vi "Config files dialogue Window.vi"(7 "Colour":u32(colorbox)=16777225, 8 "error in (no error)":errorcluster, 9 "Caption-Left button (Cancel)":string, 10 "Caption-Right button (OK)":string, 11 "Message string":string) -> (0 "error out":errorcluster, 1 "Cancelled (Left button pressed)":bool)   [LabVIEW 2020]
doc: "Use this template to create a dialog box with event handling."
uses:
  <vilib>/Utility/miscctls.llb/LVPointTypeDef.ctl
  Global Variables/General Globals.vi
panel:
  in  "Left Button":bool
  in  "Rigth Button":bool
  out "Message":string
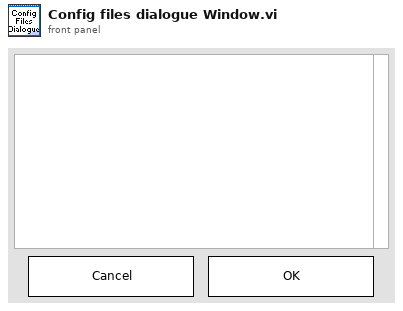
[diagram p1: front panel]
types:
  T1 = typedef "LVPointTypeDef.ctl" = cluster{"Horizontal":i16, "Vertical":i16}
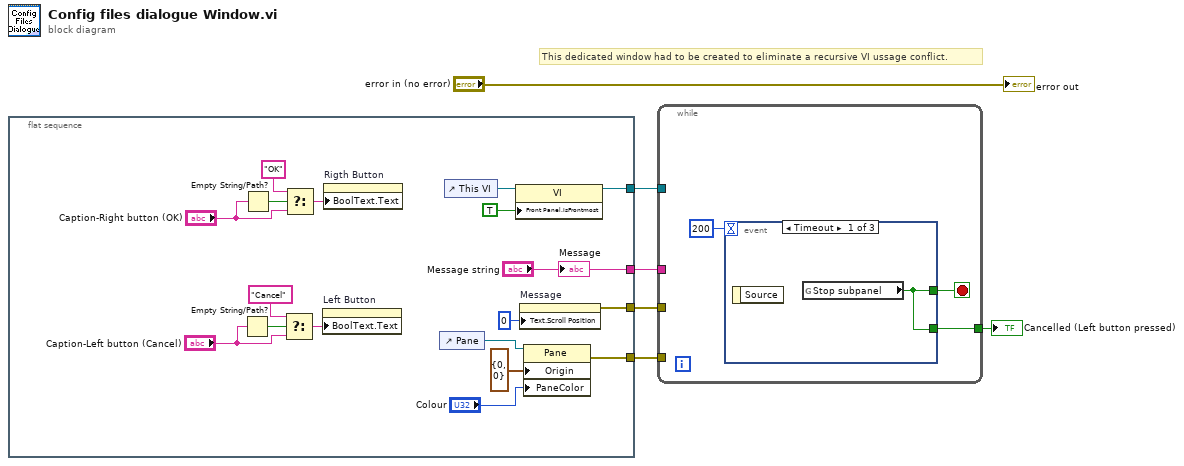
[diagram p0: block diagram]
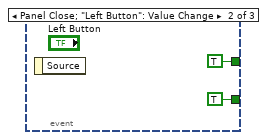
[diagram p2: hidden frame]
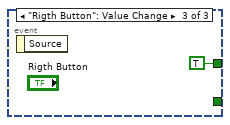
[diagram p3: hidden frame]
diagram:
  # "This dedicated window had to be created to eliminate a recursive VI ussage conflict."
  n1 = flat-sequence {
    tunnel: ["Message string"] -> w6
    tunnel: [w22] -> w5
    tunnel: [w19] -> w4
    tunnel: [w17] -> w3
    frame #0 {
      n2 = Empty String/Path?(string/path="Caption-Left button (Cancel)") -> (empty?=w10:bool)
      n3 = Empty String/Path?(string/path="Caption-Right button (OK)") -> (empty?=w14:bool)
      n4 = Select(t="Cancel", s=w10, f="Caption-Left button (Cancel)") -> (s? t:f=w9:string)
      n5 = Select(t="OK", s=w14, f="Caption-Right button (OK)") -> (s? t:f=w12:string)
      n6 = property on="Left Button" class="Bool"("BoolText.Text"=w9) -> ()  [unwired: 2 in, 2 out]
      n7 = property on="Rigth Button" class="Bool"("BoolText.Text"=w12) -> ()  [unwired: 2 in, 2 out]
      n8 = control-ref of="Pane"() -> (w16:refnum<vi>)
      n9 = control-ref of="This VI"() -> (w20:refnum<vi>)
      n10 = property on="Property Node" class="VI"(reference=w20, "Front Panel.IsFrontmost"=TRUE ("Front Panel Window:Is Frontmost")) -> (reference out=w19:refnum<vi>)  [unwired: 1 in, 1 out]
      n11 = property on="Message" class="Str"("Text.Scroll Position"=u32 0) -> (error out=w22:errorcluster)  [unwired: 2 in, 1 out]
      n12 = property class="Pane"(reference=w16, "Origin"=T1 {"Horizontal"=0, "Vertical"=0}, "PaneColor"="Colour") -> (error out=w17:errorcluster)  [unwired: 1 in, 1 out]
      "Message" <- "Message string"
    }
  }
  n13 = while {
    tunnel: w6 -> [_]
    tunnel: w5 -> [_]
    tunnel: w3 -> [_]
    tunnel: w4 -> [_]
    tunnel: [w25] -> w2
    stop <- w27 stop-if-true
    n14 = event shown="[0] Timeout" {
      selector: _ -> [_ _ _]
      dyn-events: _ -> [_ _ _]
      timeout: 200 -> [_ _ _]
      tunnel: [w28 TRUE ("Stop?") TRUE ("Stop?")] -> w27
      tunnel: [w28 TRUE ("Stop subpanel") _] -> w25
      event Timeout {
        n15 = event-data() -> ()  [unwired: 1 in, 1 out]
        n16 = global read "General Globals.vi" "Stop subpanel"() -> (w28:bool)
      }
      event Panel Close; "Left Button": Value Change {
        n17 = event-data() -> ()  [unwired: 1 in, 1 out]
      }
      event "Rigth Button": Value Change {
        n18 = event-data() -> ()  [unwired: 1 in, 1 out]
      }
    }
  }
  "Cancelled (Left button pressed)" <- w2
  "error out" <- "error in (no error)"
